vi "HWhist-SingleCurveMultiModules.vi"() -> ()   [LabVIEW 2017]
doc: "This example demonstrates how to use the Becker&Hickl LabVIEW wrapper VIs to acquire single decay curves from multiple modules in a continuous loop.\nThe SPC parameters can be adjusted during the run. The rates and status flags are continuously updated.\nIt is also possible to save the acquired data to a SDT or CSV file.\nClick this window's red X to stop this VI.\n\ninfo@becker-hickl.com"
uses:
  SPC_Wrappers/SPC_Controls/ConfigMem.ctl
  SPC_Wrappers/SPC_Controls/SPC_RatesCluster.ctl
  SPC_Wrappers/SPC_Controls/ADCResolution.ctl
  SPC_Wrappers/SPC_Controls/SPCdata.ctl
  SPC_Wrappers/SPC_Controls/StateCluster.ctl
  Example_Controls/UserInput-AllModules.ctl
  Example_Controls/UserInput-PerModules.ctl
  SPC_Wrappers/SPC_Controls/dither_range.ctl
  SPC_Wrappers/SPC_Controls/macro_time_clk.ctl
  <vilib>/Utility/file.llb/Write Delimited Spreadsheet (DBL).vi
panel:
  in  "User Input PerModules":T1[](array[typedef])=[{"sync_threshold"=-71.0, "sync_zc_level"=-5.0, "sync_freq_div"=1, "cfd_limit_low"=-50.0, "cfd_zc_level"=9.8}] {"sync_freq_div" items=["1"=1, "2"=2, "4"=4]; "cfd_zc_level" min=-96 max=96 step=0.1 format="%#_3g"; "cfd_limit_low" min=-500 max=0 step=0.1 format="%#_3g"; "sync_zc_level" min=-96 max=96 step=0.1 format="%#_3g"; "sync_threshold" min=-500 max=-20 step=0.1 format="%#_3g"}
  in  "User Input AllModules":T2={"tac_range"=50.0, "tac_gain"=3, "tac_offset"=12.0, "tac_limit_high"=96.0, "tac_limit_low"=4.0, "collect_time"=2.0} {"tac_limit_high" min=0 max=100 step=0.1; "collect_time" min=1e-07 max=100000 step=0.001; "tac_offset" min=0 max=100 step=0.1; "tac_gain" min=1 max=15 step=1; "tac_range" format="%^#_6g"}
  in  "ActiveModule":i32[](listbox)
  in  "Init":bool
  out "SPC_State":T3[](array[typedef])
  out "SPCdata":T4
  in  "TO":i32=-1
  in  "RepeatMeas":bool
  in  "SingleMeas":bool
  out "DLL Path":path=path "C:/Program Files (x86)/BH/SPCM/DLL/spcm32x64.dll"
  out "Data":u16[][](graph)
  in  "Save Data As":enum32{"SDT", "CSV"}(radio)
  in  "SaveData":bool
  in  "Name Of File":string="IRF"
  in  "SavingFolder":path=path "C:/temp"
  in  "No of Routing Channels":i16(ring)=1 items=["1"=1, "2"=2, "3"=3, "4"=4, "5"=5, "6"=6, "7"=7, "8"=8, "9"=9, "10"=10, "11"=11, "12"=12, "13"=13, "14"=14, "15"=15, "16"=16]
  in  "ADC Resolution":T5=12 items=["1"=0, "4"=2, "16"=4, "64"=6, "256"=8, "1024"=10, "4096"=12]
  out "Mod No":i16[](array[numeric])
  out "SPC_RatesCluster":T6[](array[typedef]) {"Sync" scale=0.0..6000000.0; "ADC" scale=0.0..1000000.0; "TAC" scale=0.0..1000000.0; "CFD" scale=0.0..1000000.0}
  out "SPC memory config":T7[](array[typedef]) {"Frames Per Page" min=1 step=1; "Maxpage" min=1; "Blocks Per Frame" min=1 step=1}
  in  "StopVi":bool=TRUE
  # "This example demonstrates how to use the Becker&Hickl LabVIEW wrapper VIs to acquire single decay curves from multiple modules in a continuous loop.\nThe SPC parameters can be adjusted during the run. The rates and status flags are continuously updated.\nIt is also possible to save the acquired data to a SDT or CSV file.\nClick this window's red X to stop this VI."
  # "CFD"
  # "(start)"
  # "SYNC"
  # "(stop)"
  # "threshold(LL)"
  # "zero cross(ZC)"
  # "TAC / Time Range"
  # "range"
  # "gain"
  # "offset"
  # "limit high"
  # "limit low"
  # "Collection Time"
  # "See Tip-Strip for details"
  # "(c) 2022 Becker & Hickl GmbH\n     ALL RIGHTS RESERVED."
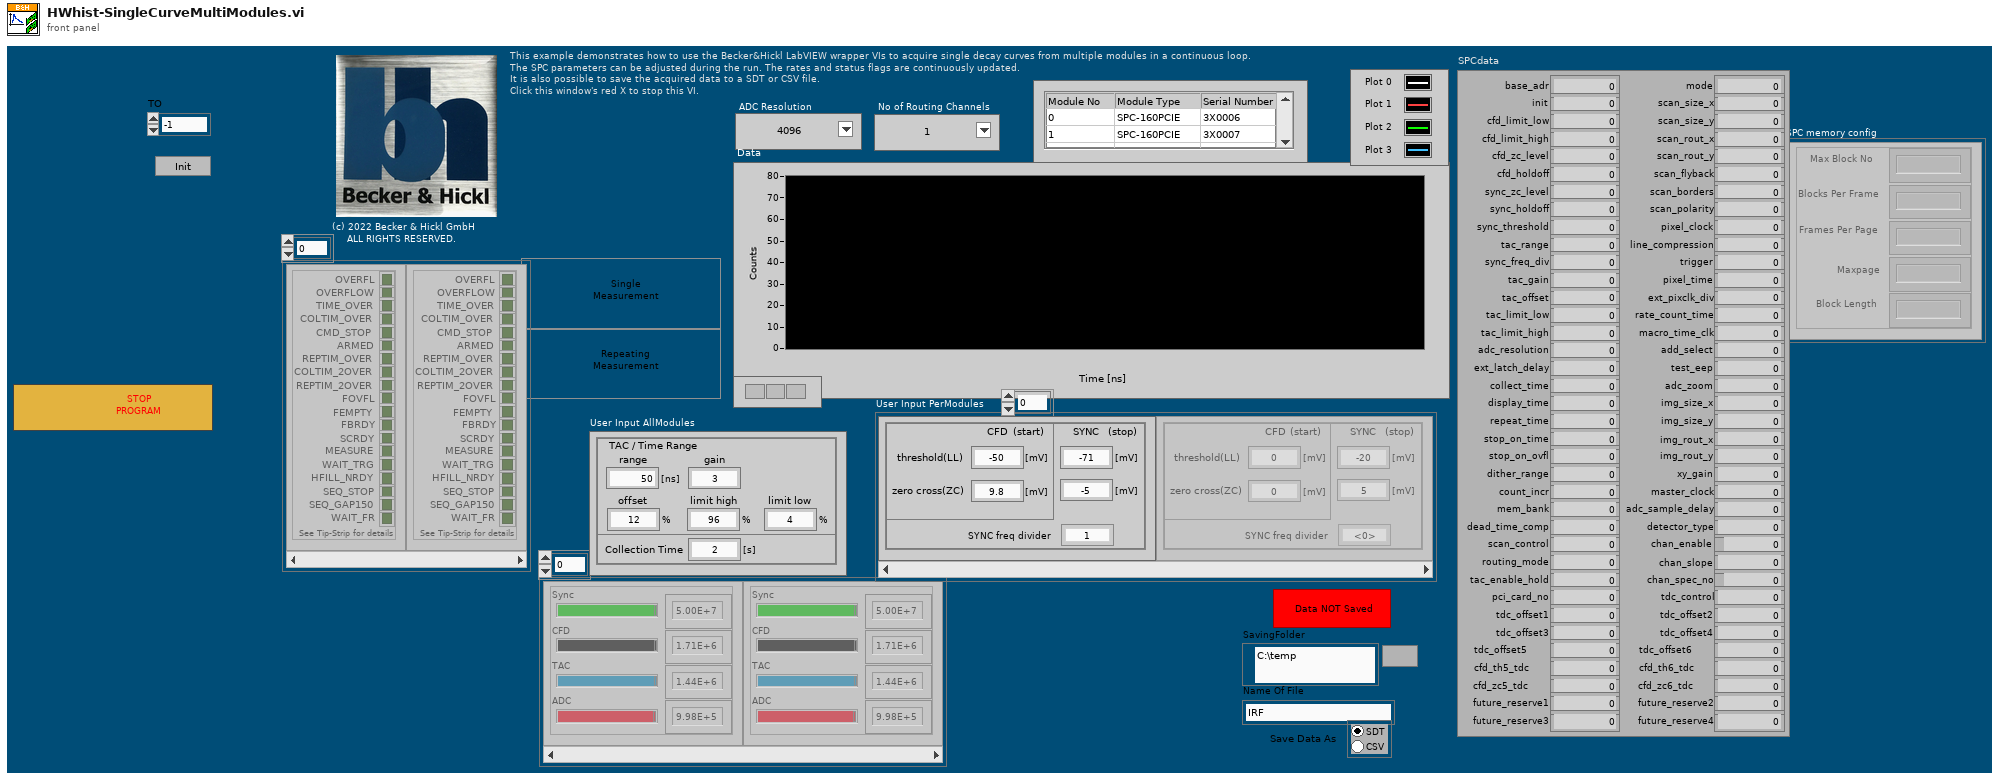
[diagram p1: front panel]
types:
  T1 = typedef "UserInput-PerModules.ctl" = cluster{"sync_threshold":sgl, "sync_zc_level":sgl, "sync_freq_div":i16, "cfd_limit_low":sgl, "cfd_zc_level":sgl}
  T2 = typedef "UserInput-AllModules.ctl" = cluster{"tac_range":sgl, "tac_gain":i16, "tac_offset":sgl, "tac_limit_high":sgl, "tac_limit_low":sgl, "collect_time":sgl}
  T3 = typedef "StateCluster.ctl" = cluster{"OVERFL":bool, "OVERFLOW":bool, "TIME_OVER":bool, "COLTIM_OVER":bool, "CMD_STOP":bool, "ARMED":bool, "REPTIM_OVER":bool, "COLTIM_2OVER":bool, "REPTIM_2OVER":bool, "FOVFL":bool, "FEMPTY":bool, "FBRDY":bool, "SCRDY":bool, "MEASURE":bool, "WAIT_TRG":bool, "HFILL_NRDY":bool, "SEQ_STOP":bool, "SEQ_GAP150":bool, "WAIT_FR":bool}
  T4 = typedef "SPCdata.ctl" = cluster{"base_adr":u16, "init":i16, "cfd_limit_low":sgl, "cfd_limit_high":sgl, "cfd_zc_level":sgl, "cfd_holdoff":sgl, "sync_zc_level":sgl, "sync_holdoff":sgl, "sync_threshold":sgl, "tac_range":sgl, "sync_freq_div":i16, "tac_gain":i16, "tac_offset":sgl, "tac_limit_low":sgl, "tac_limit_high":sgl, "adc_resolution":i16, "ext_latch_delay":i16, "collect_time":sgl, "display_time":sgl, "repeat_time":sgl, "stop_on_time":i16, "stop_on_ovfl":i16, "dither_range":i16, "count_incr":i16, "mem_bank":i16, "dead_time_comp":i16, "scan_control":u16, "routing_mode":u16, "tac_enable_hold":sgl, "pci_card_no":i16, "mode":u16, "scan_size_x":u32, "scan_size_y":u32, "scan_rout_x":u32, "scan_rout_y":u32, "scan_flyback":u32, "scan_borders":u32, "scan_polarity":u16, "pixel_clock":u16, "line_compression":u16, "trigger":u16, "pixel_time":sgl, "ext_pixclk_div":u32, "rate_count_time":sgl, "macro_time_clk":i16, "add_select":i16, "test_eep":i16, "adc_zoom":i16, "img_size_x":u32, "img_size_y":u32, "img_rout_x":u32, "img_rout_y":u32, "xy_gain":i16, "master_clock":i16, "adc_sample_delay":i16, "detector_type":i16, "chan_enable":u32, "chan_slope":u32, "chan_spec_no":u32, "tdc_control":u32, "tdc_offset1":sgl, "tdc_offset2":sgl, "tdc_offset3":sgl, "tdc_offset4":sgl, "tdc_offset5":sgl, "tdc_offset6":sgl, "cfd_th5_tdc":sgl, "cfd_th6_tdc":sgl, "cfd_zc5_tdc":sgl, "cfd_zc6_tdc":sgl, "future_reserve1":u64, "future_reserve2":u64, "future_reserve3":u64, "future_reserve4":u64}
  T5 = typedef "ADCResolution.ctl" = i16
  T6 = typedef "SPC_RatesCluster.ctl" = cluster{"Sync":sgl, "CFD":sgl, "TAC":sgl, "ADC":sgl}
  T7 = typedef "ConfigMem.ctl" = cluster{"Max Block No":i32, "Blocks Per Frame":i32, "Frames Per Page":i32, "Maxpage":i32, "Block Length":i32}
  T8 = typedef "macro_time_clk.ctl" = enum16{"25ns", "Sync", "1/2 Sync", "1/4 Sync", "1/8 Sync"}
  T9 = typedef "dither_range.ctl" = i16
  T10 = enum8{"Enabled", "Disabled", "Disabled and Grayed Out"}
  T11 = typedef "SPCModInfo.ctl" = cluster{"Module Type":T12, "Bus Number":i16, "Slot Number":i16, "in Use":i16, "Init Status":i16, "Base I/O Addr":u16}
  T12 = typedef "ModuleType.ctl" = i16
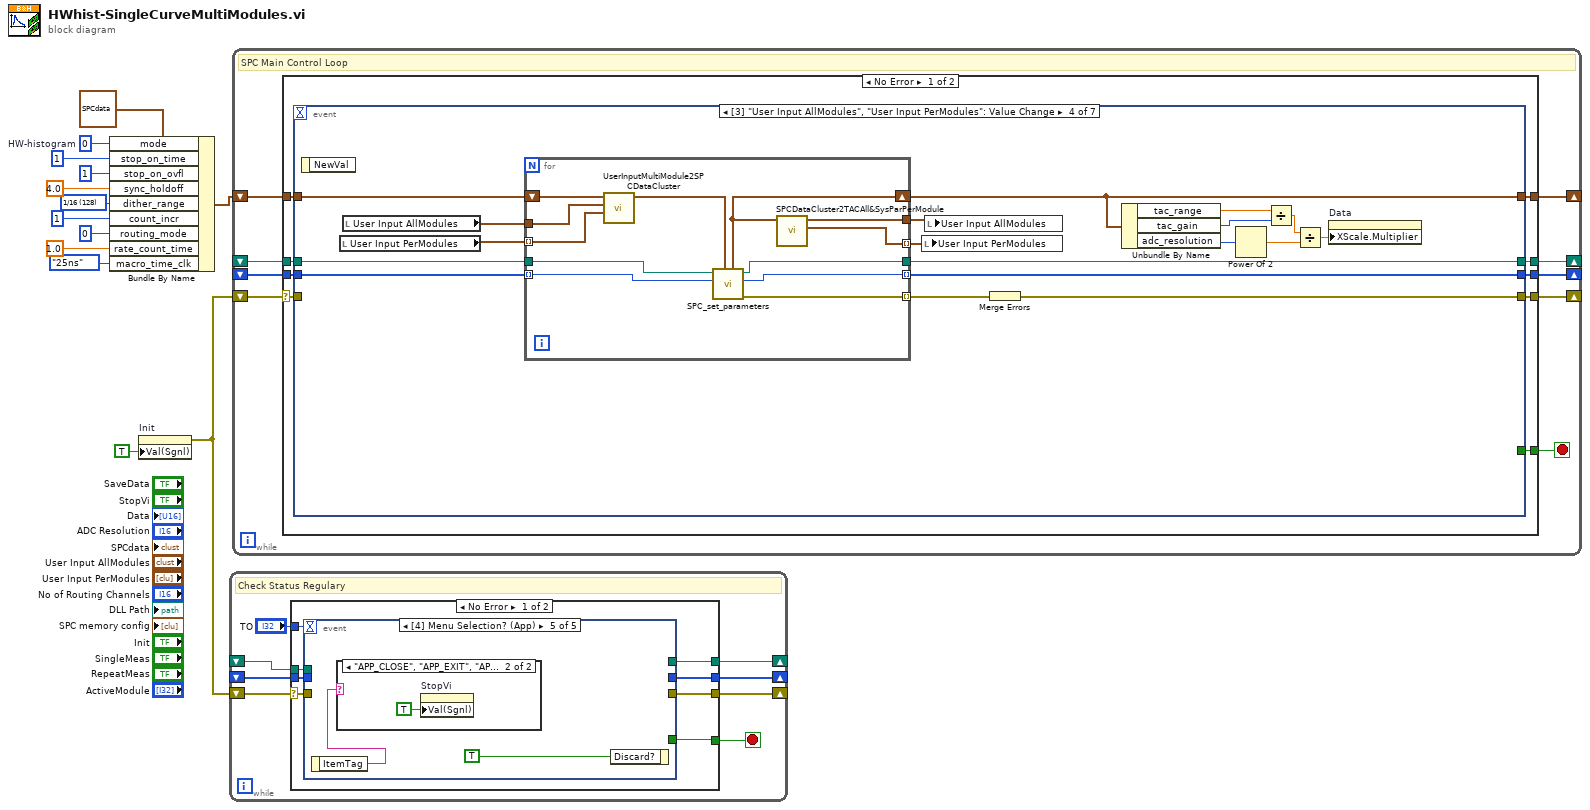
[diagram p0: block diagram]
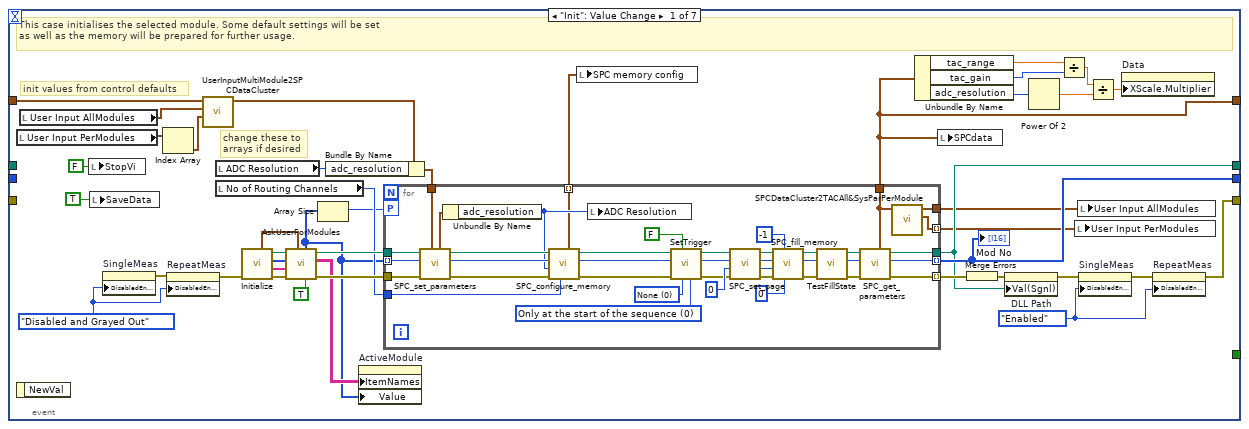
[diagram p2: hidden frame]
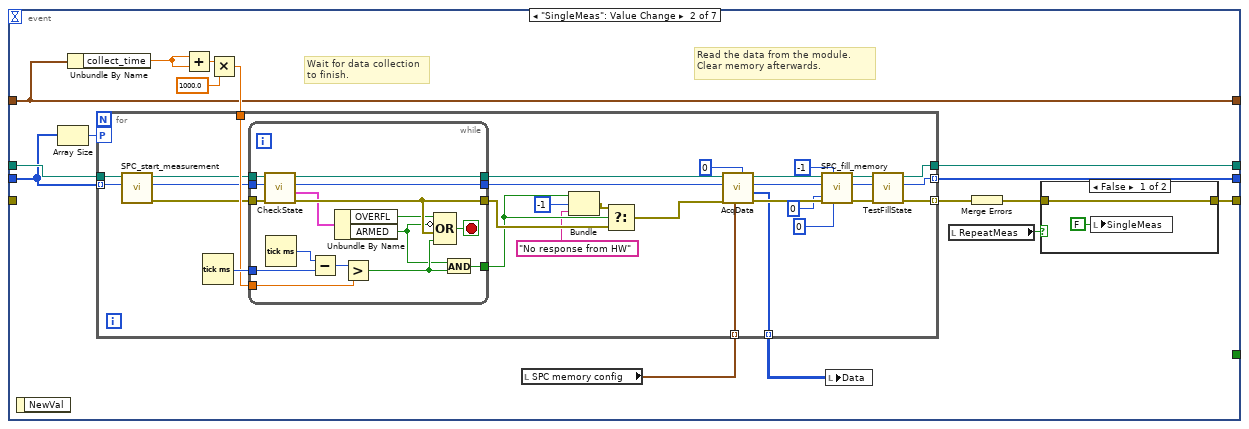
[diagram p3: hidden frame]
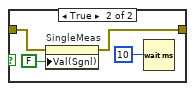
[diagram p4: hidden frame]
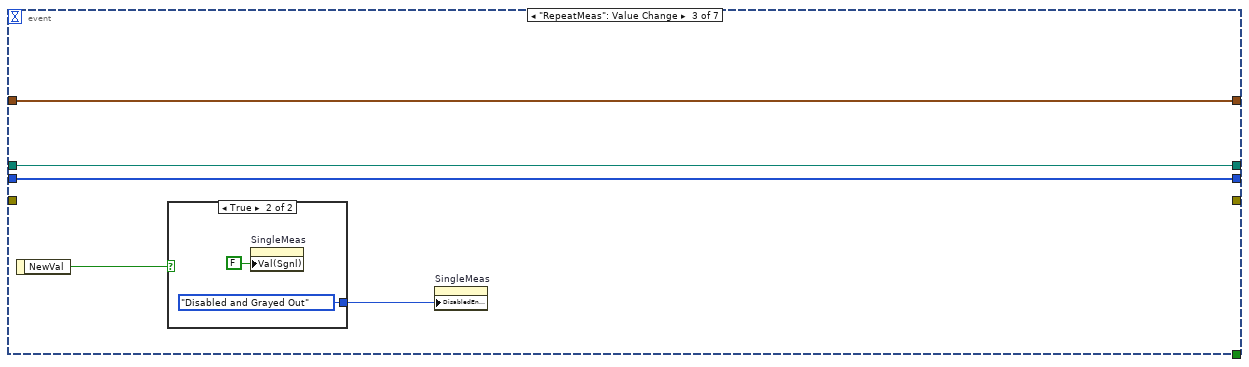
[diagram p5: hidden frame]
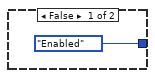
[diagram p6: hidden frame]
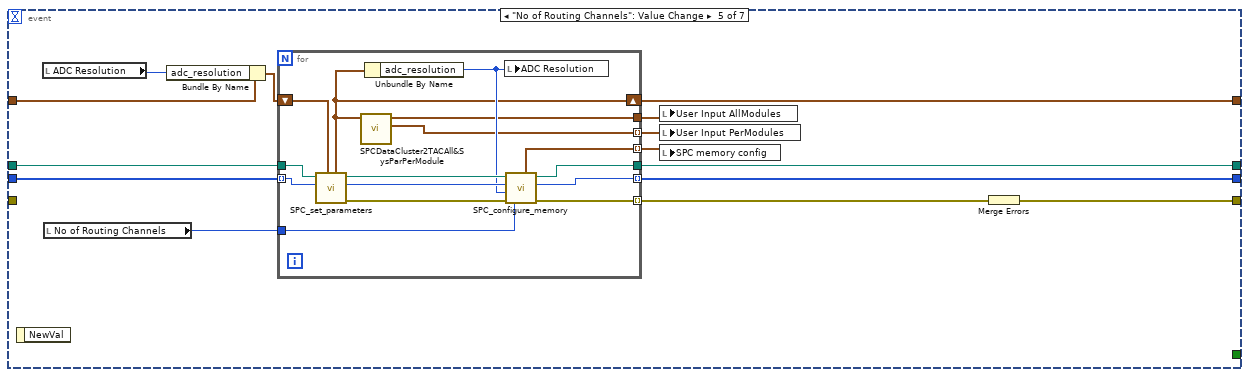
[diagram p7: hidden frame]
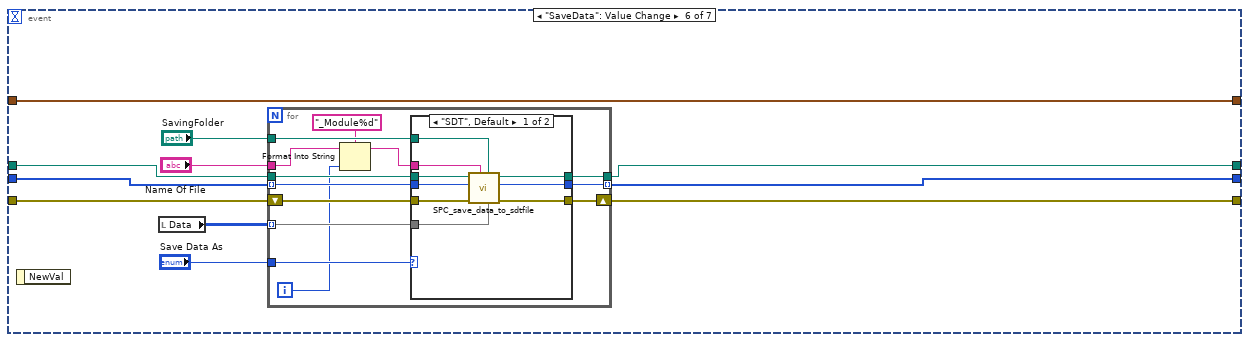
[diagram p8: hidden frame]
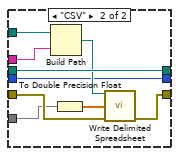
[diagram p9: hidden frame]
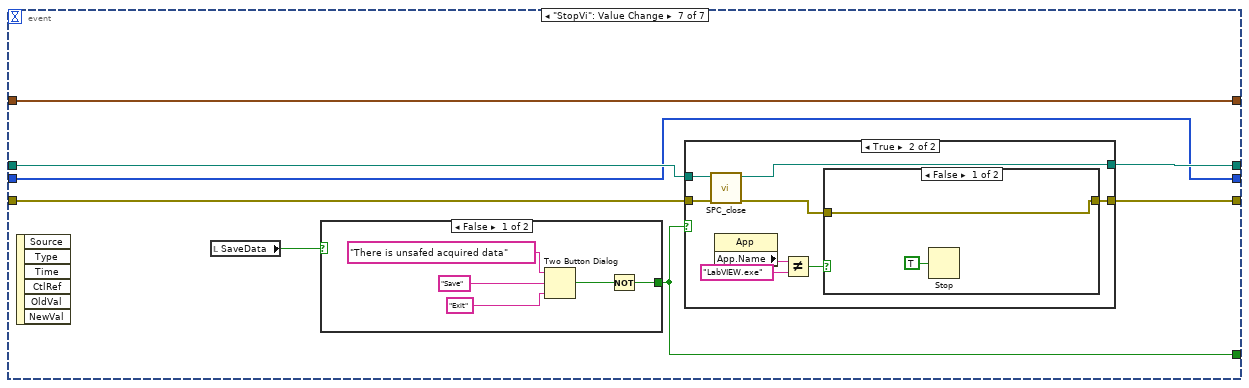
[diagram p10: hidden frame]
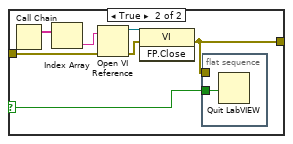
[diagram p12: hidden frame]
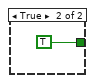
[diagram p13: hidden frame]
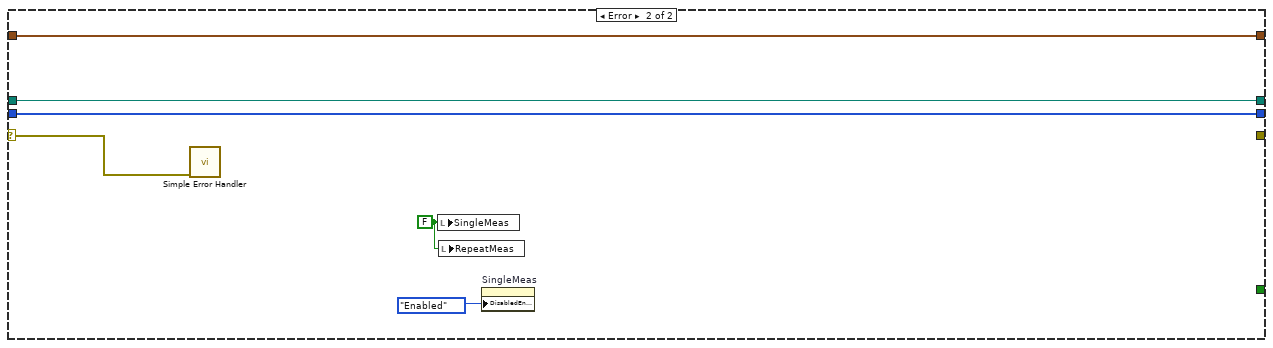
[diagram p14: hidden frame]
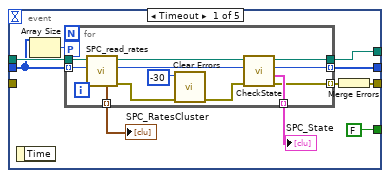
[diagram p15: hidden frame]
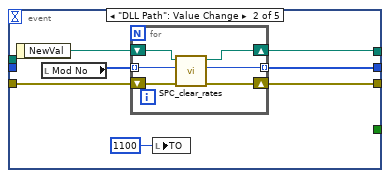
[diagram p16: hidden frame]
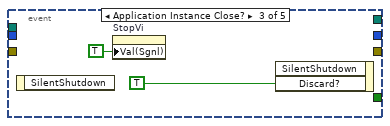
[diagram p17: hidden frame]
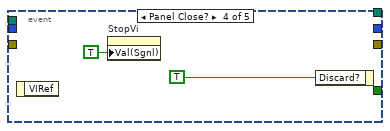
[diagram p18: hidden frame]
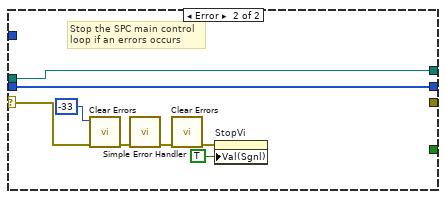
[diagram p20: hidden frame]
diagram:
  w2 = T9 128 items=["0"=0, "1/64"=32, "1/32"=64, "1/16"=128, "1/8"=256] ("DithRange")
  w11 = u16 0  # HW-histogram
  n1 = Bundle By Name(cluster=T4 {"base_adr"=896, "init"=0, "cfd_limit_low"=5.0, "cfd_limit_high"=80.0, "cfd_zc_level"=0.0, "cfd_holdoff"=5.0, "sync_zc_level"=0.0, "sync_holdoff"=4.0, "sync_threshold"=-20.0, "tac_range"=50.0, "sync_freq_div"=1, "tac_gain"=1, "tac_offset"=0.0, "tac_limit_low"=10.0, "tac_limit_high"=80.0, "adc_resolution"=10, "ext_latch_delay"=0, "collect_time"=0.01, "display_time"=1.0, "repeat_time"=10.0001, "stop_on_time"=1, "stop_on_ovfl"=1, "dither_range"=0, "count_incr"=1, "mem_bank"=0, "dead_time_comp"=1, "scan_control"=61440, "routing_mode"=0, "tac_enable_hold"=10.0, "pci_card_no"=-1, "mode"=0, "scan_size_x"=1, "scan_size_y"=1, "scan_rout_x"=1, "scan_rout_y"=1, "scan_flyback"=0, "scan_borders"=0, "scan_polarity"=0, "pixel_clock"=0, "line_compression"=1, "trigger"=0, "pixel_time"=5e-08, "ext_pixclk_div"=1, "rate_count_time"=1.0, "macro_time_clk"=0, "add_select"=0, "test_eep"=0, "adc_zoom"=0, "img_size_x"=1, "img_size_y"=1, "img_rout_x"=1, "img_rout_y"=1, "xy_gain"=1, "master_clock"=0, "adc_sample_delay"=0, "detector_type"=1, "chan_enable"=4191231, "chan_slope"=0, "chan_spec_no"=34835, "tdc_control"=0, "tdc_offset1"=0.0, "tdc_offset2"=0.0, "tdc_offset3"=0.0, "tdc_offset4"=0.0, "tdc_offset5"=0.0, "tdc_offset6"=0.0, "cfd_th5_tdc"=0.0, "cfd_th6_tdc"=0.0, "cfd_zc5_tdc"=0.0, "cfd_zc6_tdc"=0.0, "future_reserve1"=0, "future_reserve2"=0, "future_reserve3"=0, "future_reserve4"=0} ("SPCdata In"), "mode"=w11, "stop_on_time"=i16 1 ("Stop on Time"), "stop_on_ovfl"=i16 1 ("Stop on Overflow"), "sync_holdoff"=sgl 4.0, "dither_range"=w2, "count_incr"=i16 1 ("Count Increment"), "routing_mode"=u16 0 ("Routing Mode"), "rate_count_time"=sgl 1.0 ("CFD ZC Level [mV]"), "macro_time_clk"=macro_time_clk."25ns") -> (w3:T4)
  n2 = property on="Init" class="Bool (strict)"("Val(Sgnl)"=TRUE ("Value (Signaling)")) -> (error out=w13:errorcluster)  [unwired: 2 in, 1 out]
  n3 = while {
    shift-right: [w20] -> _
    shift-left: w13 -> [w21]
    shift-right: [w17] -> _
    shift-left: _ -> [w18]
    shift-right: [w15] -> _
    shift-left: _ -> [w19]
    stop <- w14 stop-if-true
    # "Check Status Regulary"
    n4 = case shown="No Error" w21 {
      selector: w21 -> [w29 w75]
      tunnel: [w28 _] -> w20
      tunnel: w19 -> [w27 w78]
      tunnel: w18 -> [w26 w79]
      tunnel: [w25 w79] -> w17
      tunnel: "TO" -> [w24 _]
      tunnel: [w23 w78] -> w15
      tunnel: [w22 _] -> w14
      frame No Error {
        n5 = event shown="[4] Menu Selection? (App)" {
          selector: _ -> [_ _ _ _ _]
          dyn-events: _ -> [_ _ _ _ _]
          timeout: w24 -> [_ _ _ _ _]
          tunnel: w29 -> [_ w58 _ _ _]
          tunnel: [w32 w57 _ _ _] -> w28
          tunnel: w27 -> [w31 _ _ _ _]
          tunnel: w26 -> [w39 _ _ _ _]
          tunnel: [w34 w54 _ _ _] -> w25
          tunnel: [w35 w53 _ _ _] -> w23
          tunnel: [FALSE ("Sync OK") _ _ _ _] -> w22
          event Timeout {
            n6 = event-data() -> ()  [unwired: 1 in, 1 out]
            n7 = Array Size(array=w31) -> (size(s)=w30:i32)
            n8 = for {
              tunnel: w31 -> [w49] mode=indexing
              tunnel: w39 -> [w48]
              tunnel: [w47] -> w37 mode=indexing
              tunnel: [w44] -> w35 mode=indexing
              tunnel: [w41] -> w34
              tunnel: [w40] -> w33 mode=indexing
              workers-P: w30 -> [_]
              tunnel: [w45] -> w36 mode=indexing
              n9 = call "SPC_read_rates.vi"("Module No"=w49, "DLL Path"=w48) -> ("Error Out"=w51:errorcluster, "Module No"=w43:i16, "DLL Path"=w42:path, "SPC_RatesCluster"=w40:T6)  [unwired: 6 in]
              n10 = call <vilib>:"Clear Errors.vi"("error in (no error)"=w51, "specific error code to clear (0: all)"=-30) -> ("error out"=w46:errorcluster)  [unwired: 4 in, 1 out]
              n11 = call "CheckState.vi"("Error In"=w46, "Module No."=w43, "DLL Path"=w42) -> ("Error Out"=w45:errorcluster, "SPC_StateCluster"=w47:T3, "Module No."=w44:i16, "DLL Path"=w41:path)  [unwired: 4 in, 1 out]
            }
            "SPC_RatesCluster" <- w33
            "SPC_State" <- w37
            n12 = Merge Errors(w36) -> (w32:errorcluster)
          }
          event "DLL Path": Value Change {
            n13 = event-data() -> ("NewVal"=w55:path)  [unwired: 1 in]
            n14 = local read "Mod No"() -> (w56:i16[])
            n15 = for {
              tunnel: w56 -> [w62] mode=indexing
              tunnel: [w59] -> w53 mode=indexing
              shift-right: [w63] -> w57
              shift-left: w58 -> [w64]
              shift-right: [w60] -> w54
              shift-left: w55 -> [w61]
              n16 = call "SPC_clear_rates.vi"("Error In"=w64, "Module no"=w62, "DLL Path"=w61) -> ("Error Out"=w63:errorcluster, "Module  No"=w59:i16, "DLL Path"=w60:path)  [unwired: 6 in]
            }
            n17 = local write "TO"(1100 ("milliseconds to wait")) -> ()
          }
          event Application Instance Close? {
            n18 = event-data() -> ()  [unwired: 1 in, 1 out]
            n19 = property on="StopVi" class="Bool (strict)"("Val(Sgnl)"=TRUE ("Value (Signaling)")) -> ()  [unwired: 2 in, 2 out]
            n20 = event-data("Discard?"=TRUE) -> ()  [unwired: 2 in, 1 out]
          }
          event Panel Close? {
            n21 = event-data() -> ()  [unwired: 1 in, 1 out]
            n22 = property on="StopVi" class="Bool (strict)"("Val(Sgnl)"=TRUE ("Value (Signaling)")) -> ()  [unwired: 2 in, 2 out]
            n23 = event-data("Discard?"=TRUE) -> ()  [unwired: 1 in, 1 out]
          }
          event Menu Selection? (App) {
            n24 = event-data() -> ("ItemTag"=w69:string)  [unwired: 1 in]
            n25 = case shown="\"APP_CLOSE\", \"APP_EXIT\", \"APP_STOP\"" w69 {
              frame Default {
                # "nothing to deal with"
              }
              frame "APP_CLOSE", "APP_EXIT", "APP_STOP" {
                n26 = property on="StopVi" class="Bool (strict)"("Val(Sgnl)"=TRUE ("Value (Signaling)")) -> ()  [unwired: 2 in, 2 out]
              }
            }
            n27 = event-data("Discard?"=TRUE) -> ()  [unwired: 1 in, 1 out]
          }
        }
      }
      frame Error {
        # "Stop the SPC main control\nloop if an errors occurs"
        n28 = call <vilib>:"Clear Errors.vi"("error in (no error)"=w75, "specific error code to clear (0: all)"=-33) -> ("error out"=w76:errorcluster)  [unwired: 4 in, 1 out]
        n29 = call <vilib>:"Simple Error Handler.vi"("error in (no error)"=w76) -> ("error out"=w73:errorcluster)  [unwired: 4 in, 4 out]
        n30 = call <vilib>:"Clear Errors.vi"("error in (no error)"=w73) -> ("error out"=w72:errorcluster)  [unwired: 5 in, 1 out]
        n31 = property on="StopVi" class="Bool (strict)"(error in=w72, "Val(Sgnl)"=TRUE ("Value (Signaling)")) -> ()  [unwired: 1 in, 2 out]
      }
    }
  }
  n32 = while {
    shift-right: [w81] -> _
    shift-left: w13 -> [w86]
    shift-right: [w87] -> _
    shift-left: _ -> [w84]
    shift-right: [w83] -> _
    shift-left: _ -> [w85]
    shift-right: [w82] -> _
    shift-left: w3 -> [w88]
    stop <- w80 stop-if-true
    # "SPC Main Control Loop"
    n33 = case shown="No Error" w86 {
      selector: w86 -> [w95 w395]
      tunnel: w88 -> [w97 w392]
      tunnel: [w96 w393] -> w87
      tunnel: w85 -> [w94 w394]
      tunnel: w84 -> [w93 w393]
      tunnel: [w92 w394] -> w83
      tunnel: [w91 w392] -> w82
      tunnel: [w90 _] -> w81
      tunnel: [w89 _] -> w80
      frame No Error {
        n34 = event shown="[3] \"User Input AllModules\", \"User Input PerModules\": Value Change" {
          selector: _ -> [_ _ _ _ _ _ _]
          dyn-events: _ -> [_ _ _ _ _ _ _]
          timeout: _ -> [_ _ _ _ _ _ _]
          tunnel: w97 -> [w103 w191 w249 w267 w294 w324 w363]
          tunnel: [w113 w186 w248 w272 w291 w317 w360] -> w96
          tunnel: w95 -> [_ _ _ _ _ w320 w361]
          tunnel: w94 -> [_ w180 w247 w269 w297 w314 w356]
          tunnel: w93 -> [_ w190 w248 w268 w296 w316 w359]
          tunnel: [w124 w185 w247 w270 w292 w315 w356] -> w92
          tunnel: [w117 w191 w249 w260 w298 w324 w363] -> w91
          tunnel: [w125 w187 _ w259 w287 w319 w358] -> w90
          tunnel: [_ _ _ _ _ _ w357] -> w89
          event "Init": Value Change {
            w116 = T10."Disabled and Grayed Out" ("Disabled")
            w129 = T10."Enabled" ("Disabled")
            # "init values from control defaults"
            # "change these to\narrays if desired"
            # "This case initialises the selected module. Some default settings will be set\nas well as the memory will be prepared for further usage."
            n35 = local read "User Input PerModules"() -> (w100:T1[])
            n36 = event-data() -> ()  [unwired: 1 in, 1 out]
            n37 = local read "User Input AllModules"() -> (w101:T2)
            n38 = local write "StopVi"(FALSE) -> ()
            n39 = local write "SaveData"(TRUE ("SaveData")) -> ()
            n40 = property on="SingleMeas" class="Bool (strict)"("DisabledEnum"=w116) -> (error out=w128:errorcluster)  [unwired: 2 in, 1 out]
            n41 = Index Array(array=w100) -> (element=w99:T1)  [unwired: 1 in]
            n42 = property on="RepeatMeas" class="Bool (strict)"(error in=w128, "DisabledEnum"=w116) -> (error out=w127:errorcluster)  [unwired: 1 in, 1 out]
            n43 = call "UserInputMultiModule2SPCDataCluster.vi"("User Input PerModules"=w99, "User Input AllModules"=w101, "SPCData_In"=w103) -> ("SPCData_Out"=w102:T4)  [unwired: 8 in]
            n44 = local read "ADC Resolution"() -> (w108:T5)
            n45 = local read "No of Routing Channels"() -> (w110:i16)
            n46 = call "Initialize.vi"("ErrorIn"=w127) -> ("ErrorOut"=w139:errorcluster, "SerialNumbersArray"=w138:string[], "ModuleNoArray"=w135:i16[], "DLL Path"=w114:path, "SPCModulesArray"=w126:T11[])  [unwired: 6 in]
            n47 = call "AskUserForModules.vi"("MultiModule"=TRUE, "SPCModulesArray"=w126, "Error In"=w139, "Serial Number"=w138, "ModuleNoArray"=w135, "DLL Path"=w114) -> ("Error Out"=w137:errorcluster, "ModuleListboxStrings"=w115:string[][], "DLL Path"=w136:path, "ActiveModuleNo"=w104:i16[])  [unwired: 1 in, 1 out]
            n48 = Array Size(array=w104) -> (size(s)=w105:i32)
            n49 = Bundle By Name(cluster=w102, "adc_resolution"=w108) -> (w109:T4)
            n50 = property on="ActiveModule" class="MCListbox (strict)"("ItemNames"=w115, "Value"=w104) -> ()  [unwired: 2 in, 2 out]
            n51 = for {
              tunnel: [w142] -> w117
              tunnel: w104 -> [w155] mode=indexing
              tunnel: [w158] -> w124 mode=indexing
              tunnel: w137 -> [w154]
              tunnel: [w159] -> w133 mode=indexing
              tunnel: w136 -> [w156]
              tunnel: [w157] -> w113
              tunnel: [w143] -> w111 mode=indexing
              tunnel: w110 -> [w144]
              workers-P: w105 -> [_]
              tunnel: w109 -> [w153]
              tunnel: [w141] -> w107
              tunnel: [w140] -> w106 mode=indexing
              w160 = i16 0 items=["Only at the start of the sequence"=0, "On each bank"=256, "On each curve in the bank"=768] ("Start Trigger")
              w162 = i16 0 items=["None", "Falling Edge", "Rising Edge"] ("Ext. Trigger Condition")
              n52 = call "SPC_set_parameters.vi"("SPCdata In"=w153, "Error In"=w154, "Module No."=w155, "DLL Path"=w156) -> ("Error Out"=w149:errorcluster, "Module No"=w150:i16, "DLL Path"=w151:path, "SPCdata Out"=w152:T4)  [unwired: 4 in]
              n53 = Unbundle By Name(w152) -> ("adc_resolution"=w145:i16)
              n54 = call "SPC_configure_memory.vi"("No of Routing\nChannels"=w144, "Error In"=w149, "ADC Resolution [exponent]"=w145, "Module No"=w150, "DLL Path"=w151) -> ("Error Out"=w148:errorcluster, "Module No"=w147:i16, "DLL Path"=w146:path, "SPCMemConfig"=w143:T7)  [unwired: 2 in, 1 out]
              n55 = local write "ADC Resolution"(w145) -> ()
              n56 = call "SetTrigger.vi"("Start Trigger"=w160, "Ext. Trigger Condition"=w162, "Master"=FALSE ("Master/Slave?"), "Error In"=w148, "Module No"=w147, "DLL Path"=w146) -> ("Error Out"=w164:errorcluster, "Module No"=w163:i16, "DLL Path"=w165:path)  [unwired: 3 in]
              n57 = call "SPC_set_page.vi"("Error In"=w164, "Page"=0 ("ADC resolution"), "Module No"=w163, "DLL Path"=w165) -> ("Error Out"=w172:errorcluster, "Page"=w178:i32, "Module No"=w173:i16, "DLL Path"=w174:path)  [unwired: 4 in]
              n58 = call "SPC_fill_memory.vi"("Fill Value"=u16 0 ("Fill value"), "Block to be Filled"=-1 ("Block to be filled"), "Error In"=w172, "Page"=w178, "Module No"=w173, "DLL Path"=w174) -> ("Error Out"=w175:errorcluster, "Module No"=w176:i16, "DLL Path"=w177:path)  [unwired: 2 in, 1 out]
              n59 = call "TestFillState.vi"("Error In"=w175, "Module No"=w176, "DLL Path"=w177) -> ("Error Out"=w166:errorcluster, "Module No"=w167:i16, "DLL Path"=w168:path)  [unwired: 6 in]
              n60 = call "SPC_get_parameters.vi"("Error In"=w166, "Module No"=w167, "DLL Path"=w168) -> ("Error Out"=w159:errorcluster, "Module No"=w158:i16, "DLL Path"=w157:path, "SPCdata"=w142:T4)  [unwired: 5 in]
              n61 = call "SPCDataCluster2TACAll&SysParPerModule.vi"("SPCdata In"=w142) -> ("User Input PerModules"=w140:T1, "User Input AllModules"=w141:T2)  [unwired: 9 in]
            }
            "Mod No" <- w124
            n62 = local write "SPC memory config"(w111) -> ()
            n63 = Unbundle By Name(w117) -> ("tac_range"=w122:sgl, "tac_gain"=w121:i16, "adc_resolution"=w120:i16)
            n64 = local write "SPCdata"(w117) -> ()
            n65 = Merge Errors(w133) -> (w112:errorcluster)
            n66 = property on="DLL Path" class="Path"(error in=w112, "Val(Sgnl)"=w113) -> (error out=w131:errorcluster)  [unwired: 1 in, 1 out]
            n67 = Power Of 2(x=w120) -> (2^x=w119:dbl)
            n68 = Divide(x=w122, y=w121) -> (x/y=w123:sgl)
            n69 = local write "User Input PerModules"(w106) -> ()
            n70 = local write "User Input AllModules"(w107) -> ()
            n71 = property on="SingleMeas" class="Bool (strict)"(error in=w131, "DisabledEnum"=w129) -> (error out=w130:errorcluster)  [unwired: 1 in, 1 out]
            n72 = Divide(x=w123, y=w119) -> (x/y=w118:dbl)
            n73 = property on="Data" class="WFGraph (strict)"("XScale.Multiplier"=w118) -> ()  [unwired: 2 in, 2 out]
            n74 = property on="RepeatMeas" class="Bool (strict)"(error in=w130, "DisabledEnum"=w129) -> (error out=w125:errorcluster)  [unwired: 1 in, 1 out]
          }
          event "SingleMeas": Value Change {
            # "Wait for data collection\nto finish."
            # "Read the data from the module.\nClear memory afterwards."
            n75 = event-data() -> ()  [unwired: 1 in, 1 out]
            n76 = Array Size(array=w180) -> (size(s)=w179:i32)
            n77 = Unbundle By Name(w191) -> ("collect_time"=w181:sgl)
            n78 = Add(x=w181, y=w181) -> (x+y=w194:sgl)
            n79 = Multiply(x=w194, y=sgl 1000.0) -> (x*y=w193:sgl)
            n80 = local read "SPC memory config"() -> (w189:T7[])
            n81 = for {
              tunnel: w193 -> [w220]
              tunnel: w190 -> [w218]
              tunnel: w180 -> [w217] mode=indexing
              tunnel: w189 -> [w204] mode=indexing
              tunnel: [w203] -> w182 mode=indexing
              tunnel: [w200] -> w183 mode=indexing
              tunnel: [w199] -> w186
              tunnel: [w198] -> w185 mode=indexing
              workers-P: w179 -> [_]
              n82 = call "SPC_start_measurement.vi"("Module No"=w217, "DLL Path"=w218) -> ("Error Out"=w219:errorcluster, "Module No"=w216:i16, "DLL Path"=w215:path)  [unwired: 7 in]
              n83 = Tick Count (ms)() -> (millisecond timer value=w224:u32)
              n84 = while {
                tunnel: w215 -> [w240]
                tunnel: w216 -> [w239]
                tunnel: w219 -> [w238]
                tunnel: [w236] -> w201
                tunnel: [w235] -> w197
                tunnel: [w234] -> w221
                tunnel: w224 -> [w232]
                tunnel: [w226] -> w196
                tunnel: w220 -> [w230]
                stop <- w237 stop-if-true
                n85 = call "CheckState.vi"("Error In"=w238, "Module No."=w239, "DLL Path"=w240) -> ("Error Out"=w234:errorcluster, "SPC_StateCluster"=w229:T3, "Module No."=w235:i16, "DLL Path"=w236:path)  [unwired: 4 in, 1 out]
                n86 = Tick Count (ms)() -> (millisecond timer value=w233:u32)
                n87 = Subtract(x=w233, y=w232) -> (x-y=w227:u32)
                n88 = Unbundle By Name(w229) -> ("OVERFL"=w228:bool, "ARMED"=w225:bool)
                n89 = Greater?(x=w227, y=w230) -> (0:w231:bool)
                n90 = Compound Arithmetic op=OR(w228, invert w225, w234, w231) -> (w237:bool)
                n91 = And(x=w225, y=w231) -> (x .and. y?=w226:bool)
              }
              n92 = Bundle(w196, "Code"=-1, "Source"="No response from HW") -> (w223:cluster{bool, "Code":i32, "Source":string})  [unwired: 1 in]
              n93 = Select(t=w223, s=w196, f=w221) -> (s? t:f=w202:errorcluster)
              n94 = call "AcqData.vi"("Page No"=0, "SPC Memory Config"=w204, "Error In"=w202, "Module No"=w197, "DLL Path"=w201) -> ("Error Out"=w209:errorcluster, "SingleBlockData"=w203:u16[], "Module No"=w206:i16, "DLL Path"=w208:path)  [unwired: 2 in, 1 out]
              n95 = call "SPC_fill_memory.vi"("Fill Value"=u16 0 ("Fill value"), "Block to be Filled"=-1 ("Block to be filled"), "Error In"=w209, "Page"=0 ("Fill value"), "Module No"=w206, "DLL Path"=w208) -> ("Error Out"=w212:errorcluster, "Module No"=w213:i16, "DLL Path"=w214:path)  [unwired: 2 in, 1 out]
              n96 = call "TestFillState.vi"("Error In"=w212, "Module No"=w213, "DLL Path"=w214) -> ("Error Out"=w200:errorcluster, "Module No"=w198:i16, "DLL Path"=w199:path)  [unwired: 6 in]
            }
            n97 = local write "Data"(w182) -> ()
            n98 = local read "RepeatMeas"() -> (w188:bool)
            n99 = Merge Errors(w183) -> (w184:errorcluster)
            n100 = case shown="False" w188 {
              tunnel: w184 -> [w242 w246]
              tunnel: [w242 w245] -> w187
              frame False {
                n101 = local write "SingleMeas"(FALSE ("StartMeas")) -> ()
              }
              frame True {
                n102 = property on="SingleMeas" class="Bool (strict)"(error in=w246, "Val(Sgnl)"=FALSE ("Value (Signaling)")) -> (error out=w245:errorcluster)  [unwired: 1 in, 1 out]
                n103 = Wait (ms)(milliseconds to wait=u32 10) -> ()  [unwired: 1 out]
              }
            }
          }
          event "RepeatMeas": Value Change {
            n104 = event-data() -> ("NewVal"=w251:bool)  [unwired: 1 in]
            n105 = case shown="True" w251 {
              tunnel: [T10."Enabled" ("Disabled") T10."Disabled and Grayed Out" ("Disabled")] -> w250
              frame False {
              }
              frame True {
                n106 = property on="SingleMeas" class="Bool (strict)"("Val(Sgnl)"=FALSE ("Value (Signaling)")) -> ()  [unwired: 2 in, 2 out]
              }
            }
            n107 = property on="SingleMeas" class="Bool (strict)"("DisabledEnum"=w250) -> ()  [unwired: 2 in, 2 out]
          }
          event "User Input PerModules": Value Change {
            n108 = event-data() -> ()  [unwired: 1 in, 1 out]
            n109 = local read "User Input PerModules"() -> (w256:T1[])
            n110 = local read "User Input AllModules"() -> (w255:T2)
            n111 = for {
              tunnel: [w284] -> w272
              tunnel: [w282] -> w270 mode=indexing
              tunnel: w269 -> [w281] mode=indexing
              tunnel: w268 -> [w280]
              shift-right: [w279] -> w260
              shift-left: w267 -> [w276]
              tunnel: [w283] -> w271 mode=indexing
              tunnel: [w278] -> w258
              tunnel: [w277] -> w257 mode=indexing
              tunnel: w256 -> [w275] mode=indexing
              tunnel: w255 -> [w274]
              n112 = call "UserInputMultiModule2SPCDataCluster.vi"("User Input PerModules"=w275, "User Input AllModules"=w274, "SPCData_In"=w276) -> ("SPCData_Out"=w273:T4)  [unwired: 8 in]
              n113 = call "SPC_set_parameters.vi"("SPCdata In"=w273, "Module No."=w281, "DLL Path"=w280) -> ("Error Out"=w283:errorcluster, "Module No"=w282:i16, "DLL Path"=w284:path, "SPCdata Out"=w279:T4)  [unwired: 5 in]
              n114 = call "SPCDataCluster2TACAll&SysParPerModule.vi"("SPCdata In"=w279) -> ("User Input PerModules"=w277:T1, "User Input AllModules"=w278:T2)  [unwired: 9 in]
            }
            n115 = local write "User Input PerModules"(w257) -> ()
            n116 = local write "User Input AllModules"(w258) -> ()
            n117 = Merge Errors(w271) -> (w259:errorcluster)
            n118 = Unbundle By Name(w260) -> ("tac_range"=w265:sgl, "tac_gain"=w264:i16, "adc_resolution"=w263:i16)
            n119 = Power Of 2(x=w263) -> (2^x=w262:dbl)
            n120 = Divide(x=w265, y=w264) -> (x/y=w266:sgl)
            n121 = Divide(x=w266, y=w262) -> (x/y=w261:dbl)
            n122 = property on="Data" class="WFGraph (strict)"("XScale.Multiplier"=w261) -> ()  [unwired: 2 in, 2 out]
          }
          event "No of Routing Channels": Value Change {
            n123 = event-data() -> ()  [unwired: 1 in, 1 out]
            n124 = local read "ADC Resolution"() -> (w288:T5)
            n125 = local read "No of Routing Channels"() -> (w289:i16)
            n126 = Bundle By Name(cluster=w294, "adc_resolution"=w288) -> (w295:T4)
            n127 = for {
              tunnel: w297 -> [w313] mode=indexing
              tunnel: w296 -> [w312]
              tunnel: [w308] -> w292 mode=indexing
              tunnel: [w306] -> w291
              shift-right: [w301] -> w298
              shift-left: w295 -> [w311]
              tunnel: [w303] -> w290 mode=indexing
              tunnel: w289 -> [w304]
              tunnel: [w309] -> w293 mode=indexing
              tunnel: [w300] -> w286
              tunnel: [w299] -> w285 mode=indexing
              n128 = call "SPC_set_parameters.vi"("SPCdata In"=w311, "Module No."=w313, "DLL Path"=w312) -> ("Error Out"=w310:errorcluster, "Module No"=w307:i16, "DLL Path"=w305:path, "SPCdata Out"=w301:T4)  [unwired: 5 in]
              n129 = call "SPCDataCluster2TACAll&SysParPerModule.vi"("SPCdata In"=w301) -> ("User Input PerModules"=w299:T1, "User Input AllModules"=w300:T2)  [unwired: 9 in]
              n130 = Unbundle By Name(w301) -> ("adc_resolution"=w302:i16)
              n131 = local write "ADC Resolution"(w302) -> ()
              n132 = call "SPC_configure_memory.vi"("No of Routing\nChannels"=w304, "Error In"=w310, "ADC Resolution [exponent]"=w302, "Module No"=w307, "DLL Path"=w305) -> ("Error Out"=w309:errorcluster, "Module No"=w308:i16, "DLL Path"=w306:path, "SPCMemConfig"=w303:T7)  [unwired: 2 in, 1 out]
            }
            n133 = local write "User Input AllModules"(w286) -> ()
            n134 = local write "User Input PerModules"(w285) -> ()
            n135 = local write "SPC memory config"(w290) -> ()
            n136 = Merge Errors(w293) -> (w287:errorcluster)
          }
          event "SaveData": Value Change {
            n137 = event-data() -> ()  [unwired: 1 in, 1 out]
            n138 = local read "Data"() -> (w323:u16[][])
            n139 = for {
              tunnel: w323 -> [w337] mode=indexing
              tunnel: "Name Of File" -> [w327]
              tunnel: "Save Data As" -> [w333]
              tunnel: [w330] -> w315 mode=indexing
              tunnel: w314 -> [w329] mode=indexing
              shift-right: [w334] -> w319
              shift-left: w320 -> [w335]
              tunnel: "SavingFolder" -> [w336]
              tunnel: w316 -> [w331]
              tunnel: [w332] -> w317
              i -> [w328]
              n140 = Format Into String(format string="_Module%d", initial string=w327, w328) -> (resulting string=w326:string)  [unwired: 1 in, 1 out]
              n141 = case shown="\"SDT\", Default" w333 {
                tunnel: [w346 w354] -> w334
                tunnel: [w345 w353] -> w332
                tunnel: w331 -> [w344 w353]
                tunnel: w335 -> [w343 w355]
                tunnel: w329 -> [w342 w347]
                tunnel: w337 -> [w341 w352]
                tunnel: w336 -> [w340 w349]
                tunnel: w326 -> [w339 w350]
                tunnel: [w338 w347] -> w330
                frame "SDT", Default {
                  n142 = call "SPC_save_data_to_sdtfile.vi"("Data"=w341, "Storing Path"=w340, "SDT File Name"=w339, "Error In"=w343, "Module No"=w342, "DLL Path"=w344) -> ("Error Out"=w346:errorcluster, "Module No"=w338:i16, "DLL Path"=w345:path)  [unwired: 2 in, 1 out]
                }
                frame "CSV" {
                  n143 = Build Path(base path=w349, name or relative path=w350) -> (appended path=w351:path)
                  n144 = To Double Precision Float(number=w352) -> (double precision float=w348:dbl[])
                  n145 = call-poly <vilib>:"Write Delimited Spreadsheet.vi"("file path (dialog if empty)"=w351, "1D data"=w348, "error in (no error)"=w355) -> ("error out"=w354:errorcluster)  [unwired: 11 in, 1 out]
                }
              }
            }
          }
          event "StopVi": Value Change {
            n146 = event-data() -> ()  [unwired: 1 in, 6 out]
            n147 = local read "SaveData"() -> (w362:bool)
            n148 = case shown="False" w362 {
              tunnel: [w384 TRUE] -> w357
              frame False {
                n149 = Two Button Dialog(message="There is unsafed acquired data", 1:"Exit", 2:"Save") -> (T button?=w385:bool)
                n150 = Not(x=w385) -> (.not. x?=w384:bool)
              }
              frame True {
              }
            }
            n151 = case shown="True" w357 {
              tunnel: w359 -> [w365 w373]
              tunnel: w361 -> [w364 w372]
              tunnel: [w365 w371] -> w360
              tunnel: [w364 w369] -> w358
              frame False {
              }
              frame True {
                n152 = call "SPC_close.vi"("Error In"=w372, "DLL Path"=w373) -> ("Error Out"=w370:errorcluster, "DLL Path"=w371:path)  [unwired: 8 in]
                n153 = property class="App"() -> ("App.Name"=w368:string)  [unwired: 2 in, 2 out]
                n154 = Not Equal?(x=w368, y="LabVIEW.exe") -> (x != y?=w366:bool)
                n155 = case shown="False" w366 {
                  selector: w366 -> [_ w378]
                  tunnel: w370 -> [w375 w380]
                  tunnel: [w375 w379] -> w369
                  frame False {
                    n156 = Stop(stop? (T)=TRUE) -> ()
                  }
                  frame True {
                    n157 = Call Chain() -> (call chain=w377:string[])
                    n158 = Index Array(array=w377) -> (element=w376:string)  [unwired: 1 in]
                    n159 = Open VI Reference(vi path=w376, error in (no error)=w380) -> (vi reference=w382:refnum<vi>, error out=w381:errorcluster)  [unwired: 4 in]
                    n160 = invoke class="VI" method="FP.Close"(reference=w382, error in=w381) -> (error out=w379:errorcluster)  [unwired: 1 in, 2 out]
                    n161 = flat-sequence {
                      tunnel: w379 -> [_]
                      tunnel: w378 -> [w383]
                      frame #0 {
                        n162 = Quit LabVIEW(quit? (T)=w383) -> ()
                      }
                    }
                  }
                }
              }
            }
          }
        }
      }
      frame Error {
        w391 = FALSE ("StartMeas")
        n163 = call <vilib>:"Simple Error Handler.vi"("error in (no error)"=w395) -> ()  [unwired: 4 in, 5 out]
        n164 = local write "SingleMeas"(w391) -> ()
        n165 = local write "RepeatMeas"(w391) -> ()
        n166 = property on="SingleMeas" class="Bool (strict)"("DisabledEnum"=T10."Enabled" ("Disabled")) -> ()  [unwired: 2 in, 2 out]
      }
    }
  }
